vi "Determine Colour.vi"(8 "Error In":errorcluster, 10 "Active Input":T1, 11 "*(type *) &x":refnum<vi>) -> (0 "Error Out":errorcluster)   [LabVIEW 2024]
uses:
  Active Input.ctl
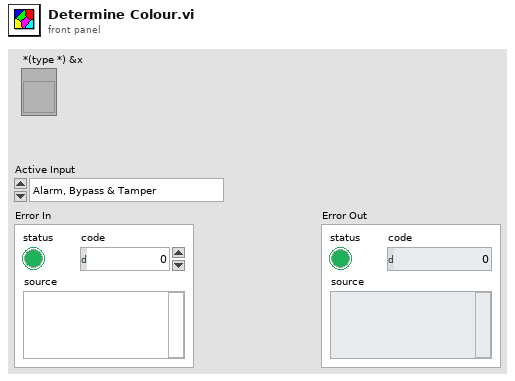
[diagram p1: front panel]
types:
  T1 = typedef "Active Input.ctl" = enum16{"Alarm, Bypass & Tamper", "Bypass & Tamper", "Alarm & Tamper", "Alarm & Bypass", "Tamper", "Bypass", "Alarm", "None"}
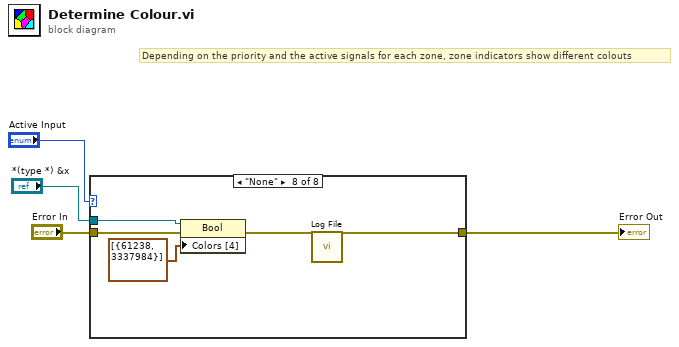
[diagram p0: block diagram]
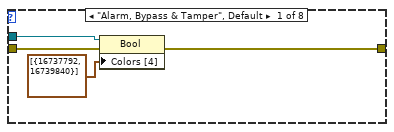
[diagram p2: hidden frame]
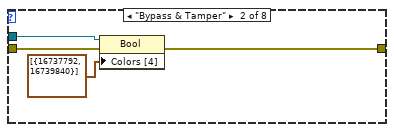
[diagram p3: hidden frame]
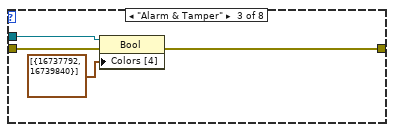
[diagram p4: hidden frame]
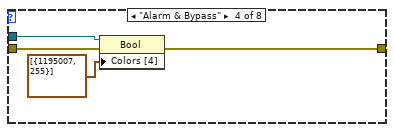
[diagram p5: hidden frame]
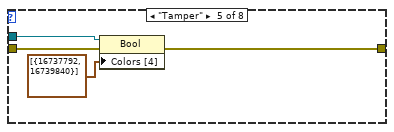
[diagram p6: hidden frame]
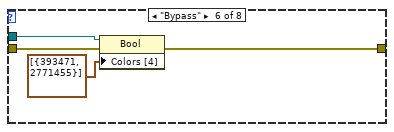
[diagram p7: hidden frame]
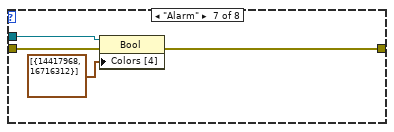
[diagram p8: hidden frame]
diagram:
  # "Depending on the priority and the active signals for each zone, zone indicators show different colouts"
  n1 = case shown="\"None\"" "Active Input" {
    tunnel: "Error In" -> [w7 w12 w16 w19 w23 w27 w32 w35]
    tunnel: [w6 w10 w15 w18 w22 w26 w31 w34] -> w3
    tunnel: "*(type *) &x" -> [w5 w9 w13 w17 w21 w25 w30 w33]
    frame "Alarm, Bypass & Tamper", Default {
      n2 = property on="Property Node" class="Bool"(reference=w5, error in=w7, "Colors [4]"=cluster{u32, u32}[] [{16737792, 16739840}]) -> (error out=w6:errorcluster)  [unwired: 1 out]
    }
    frame "Bypass & Tamper" {
      n3 = property on="Property Node" class="Bool"(reference=w9, error in=w12, "Colors [4]"=cluster{u32, u32}[] [{16737792, 16739840}]) -> (error out=w10:errorcluster)  [unwired: 1 out]
    }
    frame "Alarm & Tamper" {
      n4 = property on="Property Node" class="Bool"(reference=w13, error in=w16, "Colors [4]"=cluster{u32, u32}[] [{16737792, 16739840}]) -> (error out=w15:errorcluster)  [unwired: 1 out]
    }
    frame "Alarm & Bypass" {
      n5 = property on="Property Node" class="Bool"(reference=w17, error in=w19, "Colors [4]"=cluster{u32, u32}[] [{1195007, 255}]) -> (error out=w18:errorcluster)  [unwired: 1 out]
    }
    frame "Tamper" {
      n6 = property on="Property Node" class="Bool"(reference=w21, error in=w23, "Colors [4]"=cluster{u32, u32}[] [{16737792, 16739840}]) -> (error out=w22:errorcluster)  [unwired: 1 out]
    }
    frame "Bypass" {
      n7 = property on="Property Node" class="Bool"(reference=w25, error in=w27, "Colors [4]"=cluster{u32, u32}[] [{393471, 2771455}]) -> (error out=w26:errorcluster)  [unwired: 1 out]
    }
    frame "Alarm" {
      n8 = property on="Property Node" class="Bool"(reference=w30, error in=w32, "Colors [4]"=cluster{u32, u32}[] [{14417968, 16716312}]) -> (error out=w31:errorcluster)  [unwired: 1 out]
    }
    frame "None" {
      n9 = property on="Property Node" class="Bool"(reference=w33, error in=w35, "Colors [4]"=cluster{u32, u32}[] [{61238, 3337984}]) -> (error out=w34:errorcluster)  [unwired: 1 out]
      n10 = call "Log File.vi"() -> ()  [unwired: 12 in]
    }
  }
  "Error Out" <- w3
